vi "Untitled 2.vi"() -> ()   [LabVIEW 2020]
uses:
  <vilib>/JDP Science/JSONtext/support/Format JSON Object.vi
  <vilib>/JDP Science/JSONtext/JSONtext.lvlib
panel:
  out "length":i32
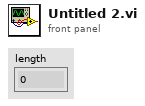
[diagram p1: front panel]
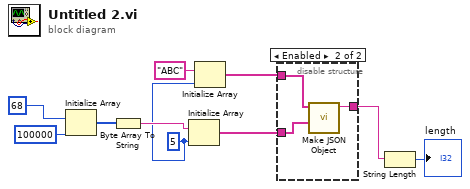
[diagram p0: block diagram]
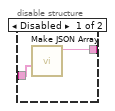
[diagram p2: hidden frame]
diagram:
  w3 = 5 ("dimension size")
  n1 = Initialize Array(u8 68 ("element"), 100000 ("dimension size")) -> (w8:u8[])
  n2 = Byte Array To String(unsigned byte array=w8) -> (string=w7:string)
  n3 = Initialize Array(w7, w3) -> (w6:string[])
  n4 = Initialize Array("ABC" ("element"), w3) -> (w1:string[])
  n5 = disable-structure shown="Enabled" {
    disable-tunnel: w6 -> [w12 w15]
    disable-tunnel: [w11 w13] -> w5
    disable-tunnel: w1 -> [_ w14]
    frame Disabled {
      n6 = call <vilib>:"Make JSON Array.vi"("JSON Elements"=w12) -> ("<JSON>"=w11:string)  [unwired: 9 in, 1 out]
    }
    frame Enabled {
      n7 = call <vilib>:"Make JSON Object.vi"("JSON Items"=w15, "Item Names"=w14) -> ("<JSON>"=w13:string)  [unwired: 8 in, 1 out]
    }
  }
  n8 = String Length(string=w5) -> (length=→"length":i32)
